vi "Fit Transform.vi"(7 "Type X":T1(ring), 8 "error in (no error)":errorcluster caption="entrée d'erreur (pas d'erreur)", 9 "y":string[][](array[string]), 10 "X":string[][](array[string]), 11 "OrdinalEncoder.lvclass":refnum<class "OrdinalEncoder.lvclass">) -> (0 "error out":errorcluster caption="sortie d'erreur", 2 "Data":T2, 3 "OrdinalEncoder.lvclass":refnum<class "OrdinalEncoder.lvclass">)   [LabVIEW 2020, in "OrdinalEncoder.lvclass"]
doc: "Fit to data, then transform it.\n\nFits transformer to X and y with optional parameters fit_params and returns a transformed version of X.\n\nReturns : \n\n- X_new : ndarray array of shape (n_samples, n_features_new)\nTransformed array."
uses:
  OrdinalEncoder.lvclass
  OrdinalEncoder.lvclass/OrdinalEncoder.ctl
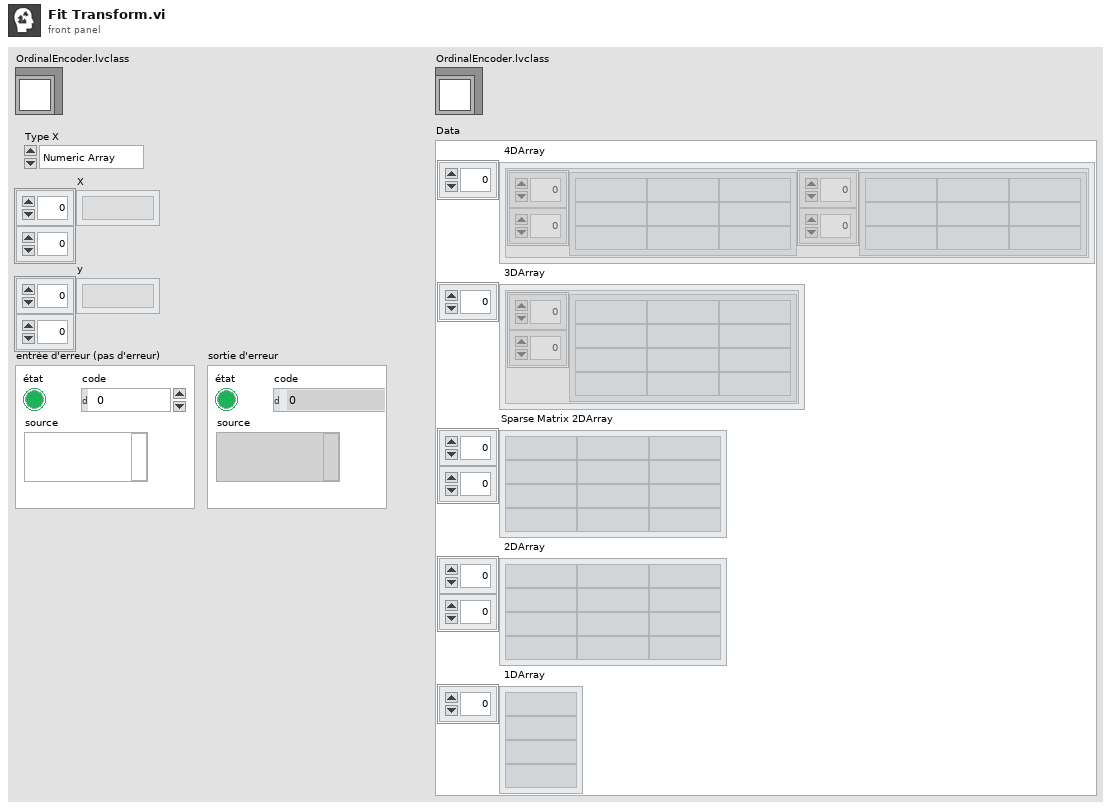
[diagram p1: front panel]
types:
  T1 = enum16{"Numeric Array", "String Array", "Sparse"}
  T2 = cluster{" 4DArray":cluster{"1":string[][], "2":string[][]}[], " 3DArray":cluster{"Tableau":string[][]}[], "Sparse Matrix 2DArray":string[][], " 2DArray":string[][], " 1DArray":string[]}
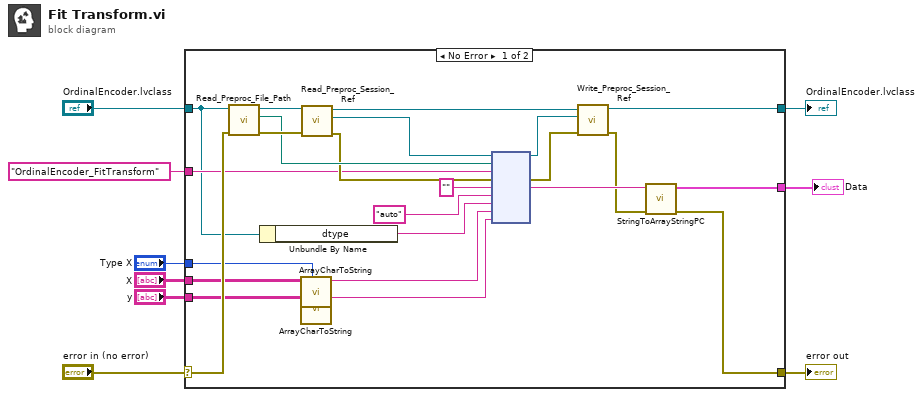
[diagram p0: block diagram]
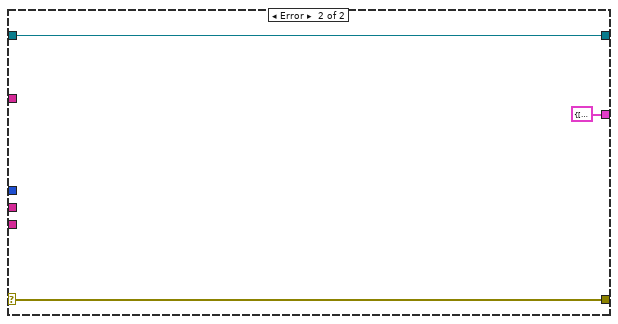
[diagram p2: hidden frame]
diagram:
  n1 = case shown="No Error" "error in (no error)" {
    selector: "error in (no error)" -> [w23 w36]
    tunnel: [w10 w36] -> w8
    tunnel: [w12 w35] -> w6
    tunnel: "OrdinalEncoder.lvclass" -> [w21 w35]
    tunnel: "OrdinalEncoder_FitTransform" ("Fonction") -> [w22 _]
    tunnel: [w11 T2 {" 4DArray"=[], " 3DArray"=[], "Sparse Matrix 2DArray"=[], " 2DArray"=[], " 1DArray"=[]} ("Data")] -> w1
    tunnel: "X" -> [w19 _]
    tunnel: "y" -> [w18 _]
    tunnel: "Type X" -> [w17 _]
    frame No Error {
      n2 = call-dynamic "Read_Preproc_File_Path.vi"("error in (no error)"=w23, "Python in"=w21) -> ("error out"=w32:errorcluster, "File_Path"=w29:path, "Python out"=w33:refnum<class "OrdinalEncoder.lvclass">)  [unwired: 7 in]
      n3 = Unbundle By Name(w21) -> ("dtype"=w24:string)
      n4 = call "ArrayCharToString.vi"("Type"=w17, "TAB"=w19) -> ("Instruction"=w16:string)  [unwired: 9 in]
      n5 = call "ArrayCharToString.vi"("TAB"=w18) -> ("Instruction"=w15:string)  [unwired: 10 in]
      n6 = call-dynamic "Read_Preproc_Session_Ref.vi"("error in (no error)"=w32, "Python in"=w33) -> ("error out"=w28:errorcluster, "Session_ref"=w30:refnum<k35>, "Python out"=w31:refnum<class "OrdinalEncoder.lvclass">)  [unwired: 7 in]
      n7 = node(w30, w29, w22, w28, "", "auto", w24, w16, w15) -> (w26:refnum<k35>, w27:errorcluster, w14:string)  [unwired: 4 in, 2 out]
      n8 = call-dynamic "Write_Preproc_Session_Ref.vi"("error in (no error)"=w27, "Session_ref"=w26, "Python in"=w31) -> ("error out"=w13:errorcluster, "Python out"=w12:refnum<class "OrdinalEncoder.lvclass">)  [unwired: 7 in]
      n9 = call "StringToArrayStringPC.vi"("sortie d'erreur"=w13, "Return value"=w14) -> ("sortie d'erreur"=w10:errorcluster, "Data"=w11:T2)  [unwired: 8 in]
    }
    frame Error {
    }
  }
  "error out" <- w8
  "OrdinalEncoder.lvclass" <- w6
  "Data" <- w1
